vi "EncoderPositionCalc.vi"(9 "PositionTarget(in)":dbl, 10 "Wheel Size(in)":dbl=4.0, 11 "EncoderCount/Revolution":dbl=4096.0) -> (3 "PostionTarget(Counts)":i32)   [LabVIEW 2017]
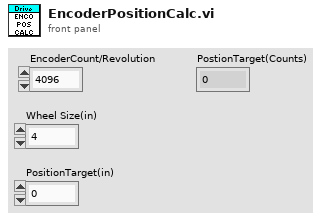
[diagram p1: front panel]
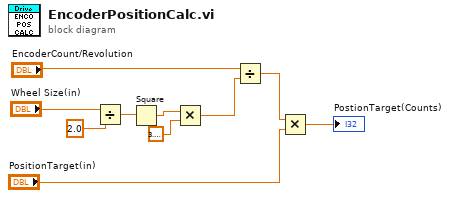
[diagram p0: block diagram]
diagram:
  n1 = Divide(x="Wheel Size(in)", y=2.0) -> (x/y=w2:dbl)
  n2 = Square(x=w2) -> (x^2=w3:dbl)
  n3 = Multiply(x=w3, y=3.141592653589793) -> (x*y=w6:dbl)
  n4 = Divide(x="EncoderCount/Revolution", y=w6) -> (x/y=w8:dbl)
  n5 = Multiply(x=w8, y="PositionTarget(in)") -> (x*y=→"PostionTarget(Counts)":dbl)
